vi "Next Runnable in Suite.vi"(8 "error in (no error)":errorcluster, 11 "LUnit Test Suite In":refnum<class "LUnit Test Suite.lvclass">) -> (0 "error out":errorcluster, 2 "Next":string, 3 "LUnit Test Suite Out":refnum<class "LUnit Test Suite.lvclass">)   [LabVIEW 2020, in "LUnit Test Suite.lvclass"]
uses:
  LUnit Test Suite.lvclass
  LUnit Test Suite.lvclass/LUnit Test Suite.ctl
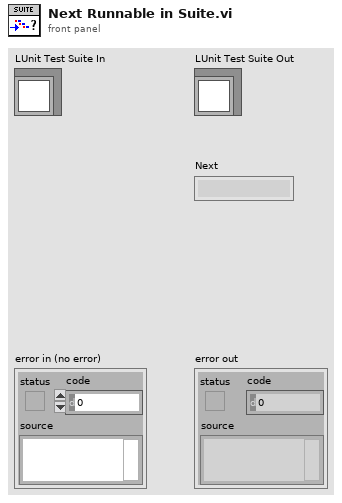
[diagram p1: front panel]
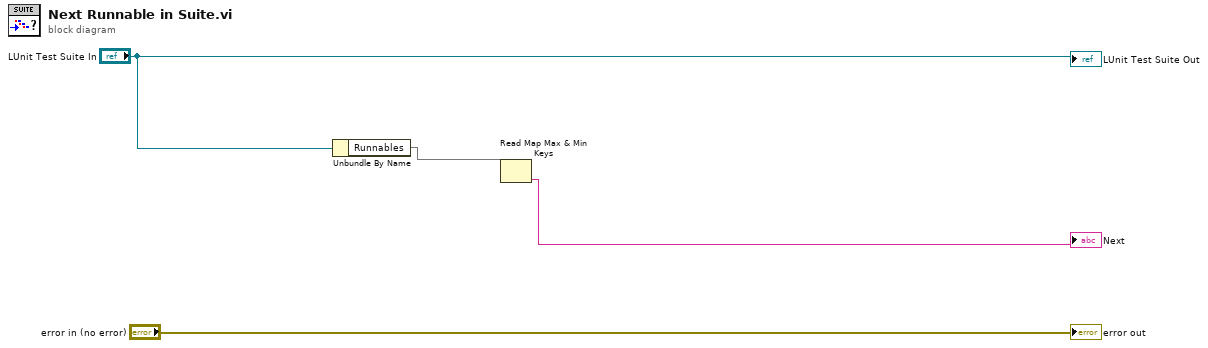
[diagram p0: block diagram]
diagram:
  n1 = Unbundle By Name("LUnit Test Suite In") -> ("Runnables"=w1:map{string, refnum<class "Runnable.lvclass">})
  n2 = Read Map Max & Min Keys(11:w1) -> (1:→"Next":string)  [unwired: 1 out]
  "error out" <- "error in (no error)"
  "LUnit Test Suite Out" <- "LUnit Test Suite In"
